vi "Create Client.vi"(8 "error in":errorcluster, 10 "Server Certificate File (.crt)":path, 11 "address":string) -> (0 "error out":errorcluster, 3 "gRPC ID Out":T1)   [LabVIEW 2021, in "CIFManagerClientWrapper.lvlib"]
uses:
  CIFManagerClientWrapper.lvlib
  <vilib>/gRPC/LabVIEW gRPC Library/Shared/grpcId.ctl
  <vilib>/gRPC/LabVIEW gRPC Library/grpc-lvsupport-release.lvlib
  CIF_Manager_client/CIF_Manager_client.lvlib
  CIFUtilities/CIFConfigurationFile/CIF Configuration File.lvlib
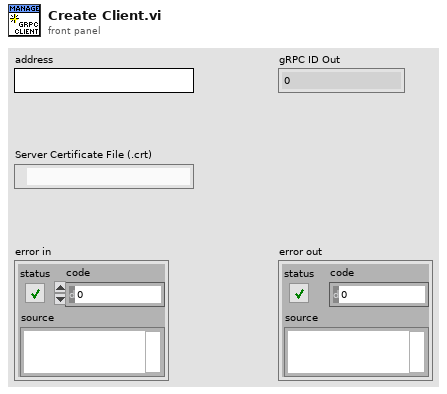
[diagram p1: front panel]
types:
  T1 = typedef "grpc-lvsupport-release.lvlib/grpcId.ctl" = u64
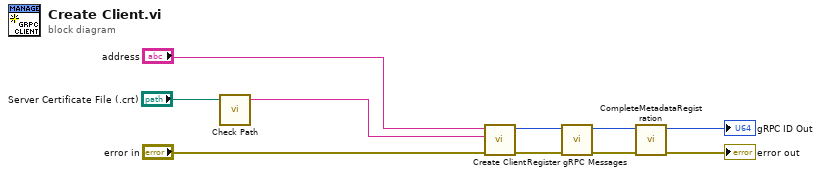
[diagram p0: block diagram]
diagram:
  n1 = call "Check Path.vi"("path"="Server Certificate File (.crt)") -> ("Path String"=w6:string)  [unwired: 3 in]
  n2 = call <vilib>:"Create Client.vi"("error in"="error in", "certificate path"=w6, "address"="address") -> ("error out"=w3:errorcluster, "ClientID out"=w4:T1)  [unwired: 7 in]
  n3 = call "Register gRPC Messages.vi"("error in (no error)"=w3, "gRPC ID"=w4) -> ("error out"=w1:errorcluster, "gRPC ID Out"=w2:T1)  [unwired: 8 in]
  n4 = call <vilib>:"CompleteMetadataRegistration.vi"("error in"=w1, "gRPC ID in"=w2) -> ("error out"=→"error out":errorcluster, "gRPC ID Out"=→"gRPC ID Out":T1)  [unwired: 8 in]
